vi "Initialize Attributes.vi"(8 "error in (no error)":errorcluster, 10 "Attribute Data":variant, 11 "PVConnection in":refnum<class "PVConnection.lvclass">) -> (0 "error out":errorcluster, 2 "Found?":bool, 3 "PVConnection out":refnum<class "PVConnection.lvclass">)   [LabVIEW 2012, in "CS++ProcessVariables.lvlib" / "PVConnection.lvclass"]
doc: "Initialize object attribute.\n\nUnique resources should be allocated elsewhere!"
uses:
  PVConnection.lvclass
  CS++BaseClasses/Base/CS++Base.lvclass
  PVConnection.lvclass/PVConnection.ctl
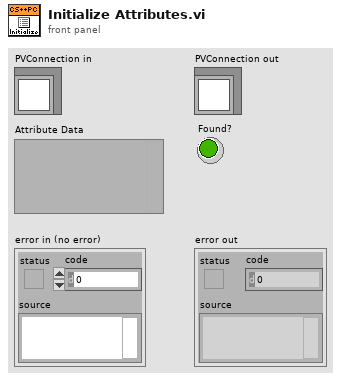
[diagram p1: front panel]
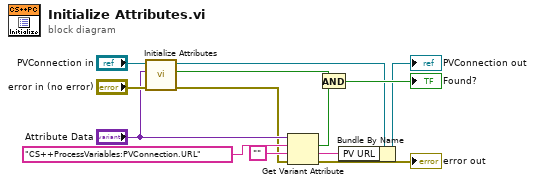
[diagram p0: block diagram]
diagram:
  n1 = call-parent "Initialize Attributes.vi"("error in (no error)"="error in (no error)", "Attribute Data"="Attribute Data", "CS++Base in"="PVConnection in") -> ("error out"=w7:errorcluster, "Found?"=w13:bool, "CS++Base out"=w3:refnum<class "PVConnection.lvclass">)  [unwired: 6 in]
  n2 = Get Variant Attribute(Variant="Attribute Data", name="CS++ProcessVariables:PVConnection.URL", default value (empty Variant)="", error in=w7) -> (found=w4:bool, value=w1:string, error out=→"error out":errorcluster)  [unwired: 1 out]
  n3 = And(x=w13, y=w4) -> (x .and. y?=→"Found?":bool)
  n4 = Bundle By Name(cluster=w3, "PV URL"=w1) -> (→"PVConnection out":refnum<class "PVConnection.lvclass">)
